vi "Labview_USB_I2C_AT24C02.vi"() -> ()   [LabVIEW 2010]
uses:
  Labview_USB_I2C_AM2321B/lib/labview_32bit/ControlI2C/Ginkgo_Driver.dll
panel:
  out "Flag(T:read;F:write)":bool=TRUE
  in  "Constant":T1={"DevType"=1, "DevIndex"=0, "I2CIndex"=0, "Addr"=0, "SubAddr"=0}
  in  "pInitConfig":T2={"MasterMode"=1, "ControlMode"=1, "AddrType"=7, "SubAddrWidth"=0, "Addr"=0, "@dummy control@"=0, "@dummy control@"=0, "ClockSpeed"=0}
  out "error out":errorcluster
  in  "Read":bool
  in  "Write":bool
  in  "Sub Addr(Hex)":u8 format="%x"
  in  "Slave Addr(Hex)":u8 format="%x"
  out "Read Data(Hex)":string
  in  "Channel Index":u16(ring) items=["0", "1"]
  in  "Speed":u32(ring)=800000 items=["800Kbps"=800000, "400Kbps"=400000, "200Kbps"=200000, "100Kbps"=100000, "50Kbps"=50000]
  in  "Write Data(Hex)":string
  in  "Device Index":u16(ring) items=["0", "1", "2", "3", "4", "5", "6", "7", "8", "9"]
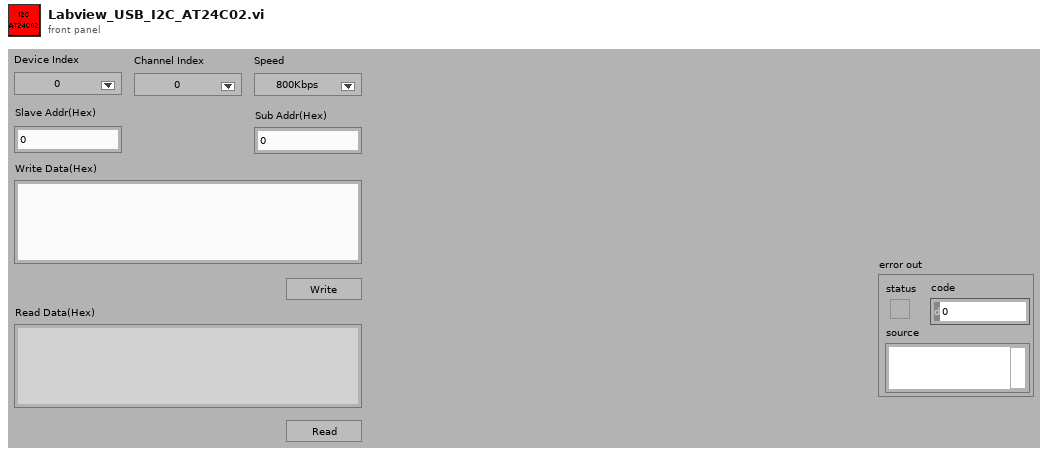
[diagram p1: front panel]
types:
  T1 = cluster{"DevType":i32, "DevIndex":i32, "I2CIndex":i32, "Addr":u16, "SubAddr":u32}
  T2 = cluster{"MasterMode":u8, "ControlMode":u8, "AddrType":u8, "SubAddrWidth":u8, "Addr":u16, "@dummy control@":i8, "@dummy control@":i8, "ClockSpeed":u32}
  T3 = enum16{"Init", "Write", "Read", "Idel", "Close", "Error"}
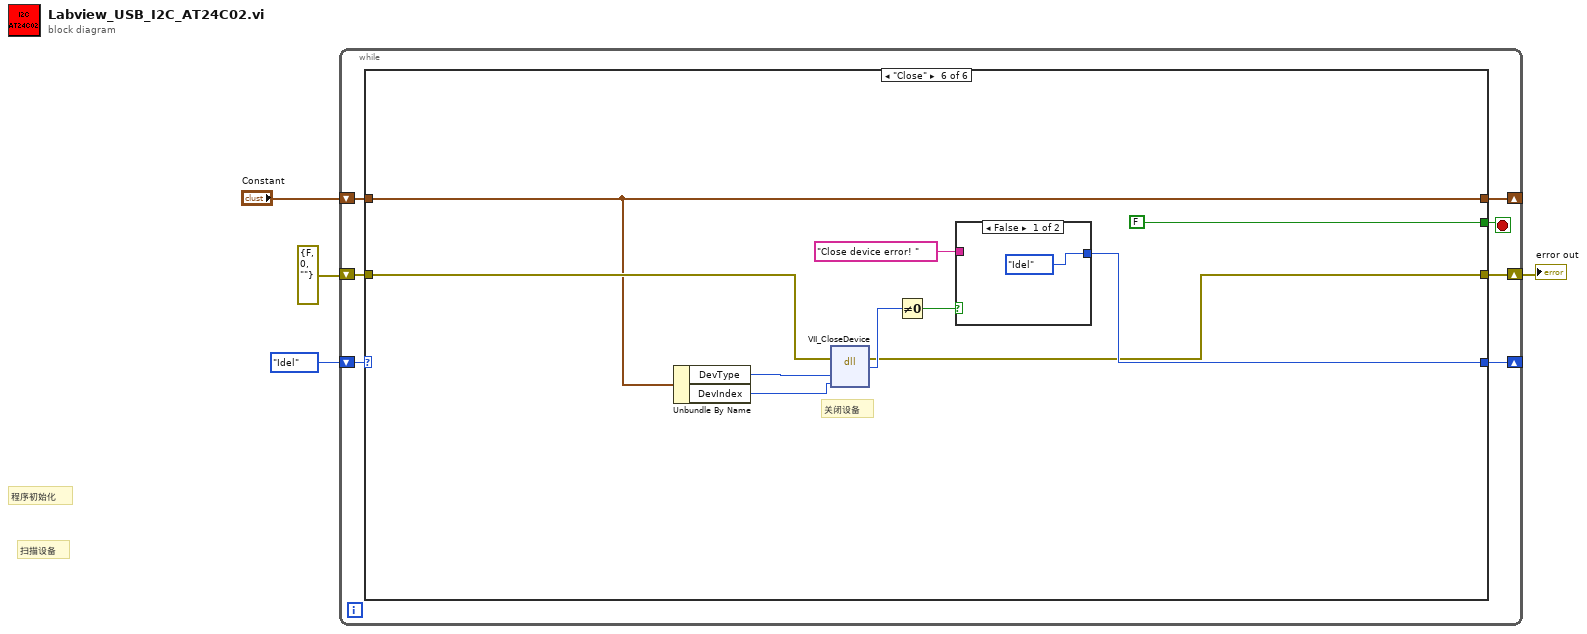
[diagram p0: block diagram]
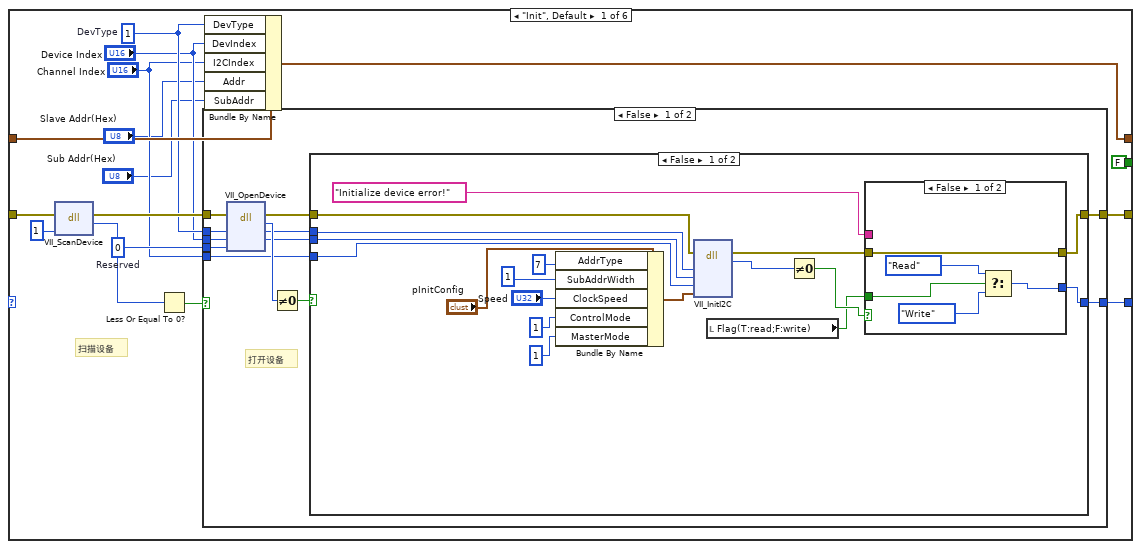
[diagram p2: hidden frame]
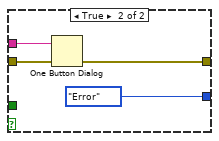
[diagram p3: hidden frame]
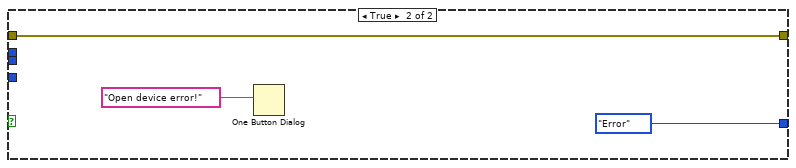
[diagram p4: hidden frame]
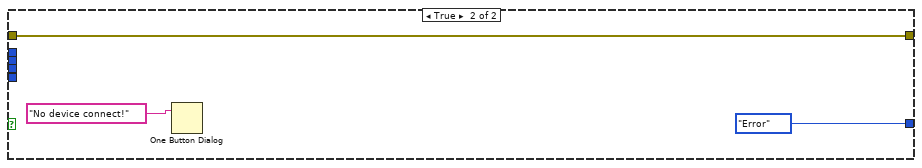
[diagram p5: hidden frame]
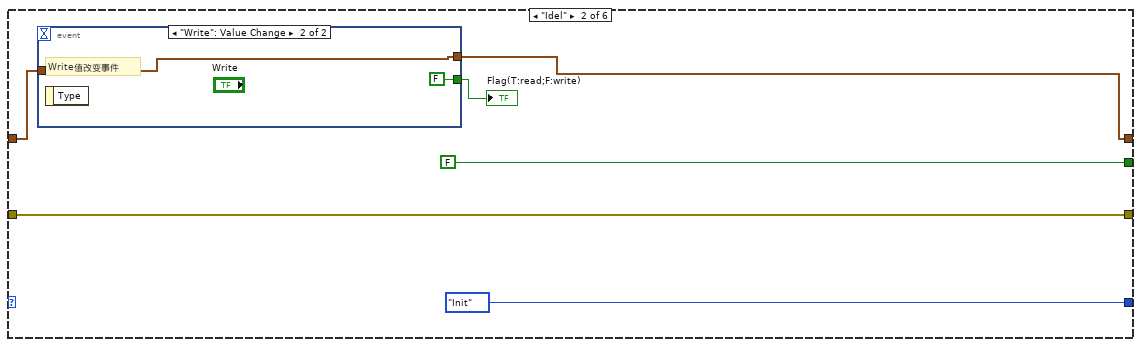
[diagram p6: hidden frame]
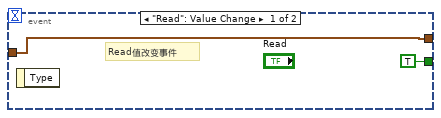
[diagram p7: hidden frame]
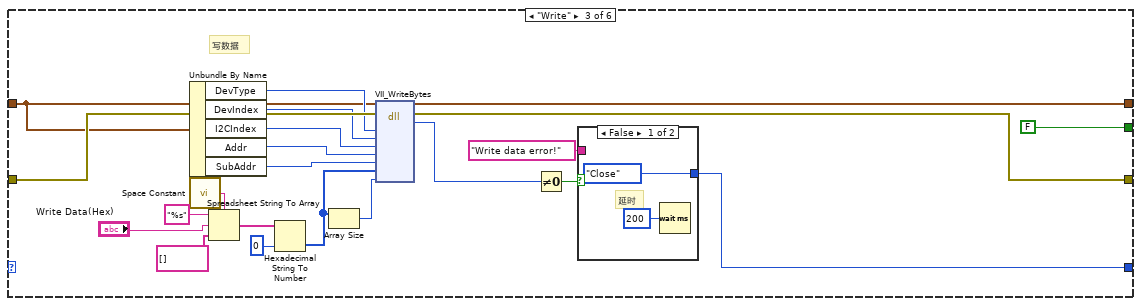
[diagram p8: hidden frame]
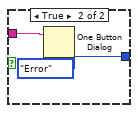
[diagram p9: hidden frame]
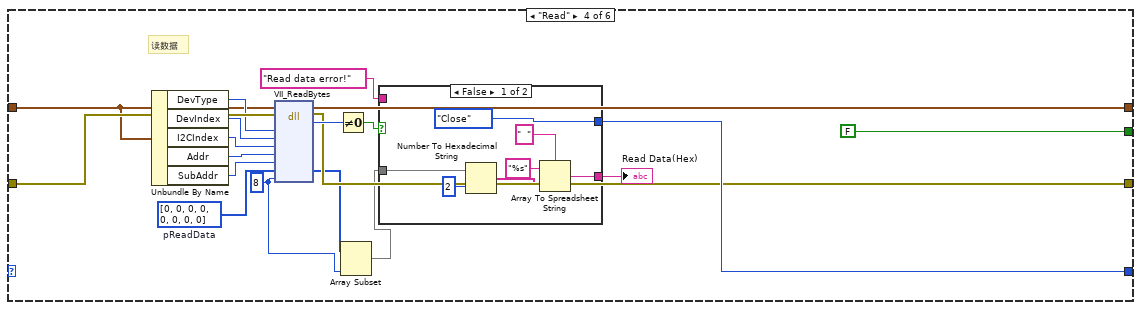
[diagram p10: hidden frame]
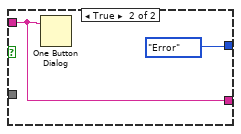
[diagram p11: hidden frame]
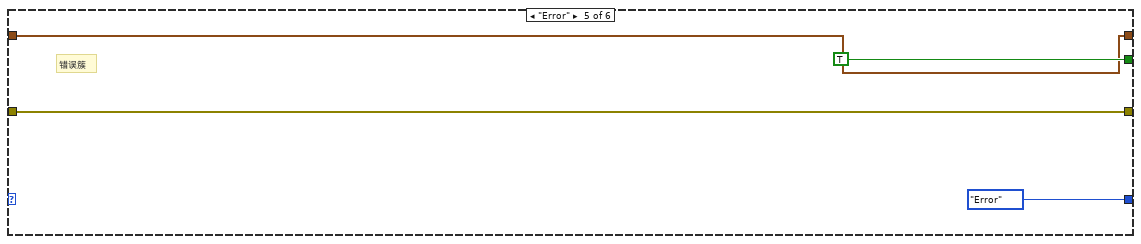
[diagram p12: hidden frame]
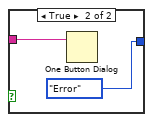
[diagram p13: hidden frame]
diagram:
  # "扫描设备"
  # "程序初始化"
  n1 = while {
    shift-right: [w11] -> _
    shift-left: T3."Idel" ("Enum") -> [w10]
    shift-right: [w8] -> w2
    shift-left: errorcluster {"status"=FALSE, "code"=0, "source"=""} ("error out") -> [w7]
    shift-right: [w5] -> _
    shift-left: "Constant" -> [w6]
    stop <- w9 stop-if-true
    n2 = case shown="\"Close\"" w10 {
      tunnel: [w19 T3."Init" ("Enum") w92 w115 T3."Error" ("Enum") w143] -> w11
      tunnel: [FALSE ("stop") FALSE ("stop") FALSE ("stop") FALSE ("stop") TRUE ("stop") FALSE ("stop")] -> w9
      tunnel: [w20 w76 w91 w114 w136 w142] -> w8
      tunnel: w7 -> [w21 w76 w101 w123 w136 w141]
      tunnel: w6 -> [w18 w75 w95 w113 w134 w140]
      tunnel: [w12 w74 w95 w113 w134 w140] -> w5
      frame "Init", Default {
        w22 = 0  # Reserved
        w17 = 1  # DevType
        # "扫描设备"
        n3 = dll-call lib="E:/Project/vt_ginkgo_examples/trunk/Labview/Ginkgo I2C/Labview_USB_I2C_AM2321B/lib/labview_32bit/ControlI2C/Ginkgo_Driver.dll" fn="VII_ScanDevice"(error in=w21, "NeedInit"=u8 1) -> (error out=w23:errorcluster, "return type"=w25:i32)  [unwired: 3 in, 1 out]
        n4 = Less Or Equal To 0?(x=w25) -> (x <= 0?=w24:bool)
        n5 = case shown="False" w24 {
          tunnel: [w33 T3."Error" ("Enum")] -> w19
          tunnel: w23 -> [w37 w70]
          tunnel: w22 -> [w36 _]
          tunnel: "Device Index" -> [w35 _]
          tunnel: w17 -> [w34 _]
          tunnel: [w29 w70] -> w20
          tunnel: "Channel Index" -> [w28 _]
          frame False {
            # "打开设备"
            n6 = dll-call lib="E:/Project/vt_ginkgo_examples/trunk/Labview/Ginkgo I2C/Labview_USB_I2C_AM2321B/lib/labview_32bit/ControlI2C/Ginkgo_Driver.dll" fn="VII_OpenDevice"(error in=w37, "DevType"=w34, "DevIndex"=w35, "Reserved"=w36) -> (error out=w32:errorcluster, "return type"=w38:i32, "DevType"=w31:i32, "DevIndex"=w30:i32)  [unwired: 3 in, 1 out]
            n7 = Not Equal To 0?(x=w38) -> (x != 0?=w39:bool)
            n8 = case shown="False" w39 {
              tunnel: [w46 T3."Error" ("Enum")] -> w33
              tunnel: w32 -> [w49 w67]
              tunnel: w31 -> [w48 _]
              tunnel: w30 -> [w47 _]
              tunnel: [w45 w67] -> w29
              tunnel: w28 -> [w44 _]
              frame False {
                n9 = Bundle By Name(cluster="pInitConfig", "AddrType"=u8 7, "SubAddrWidth"=u8 1, "ClockSpeed"="Speed", "ControlMode"=u8 1, "MasterMode"=u8 1) -> (w55:T2)
                n10 = dll-call lib="E:/Project/vt_ginkgo_examples/trunk/Labview/Ginkgo I2C/Labview_USB_I2C_AM2321B/lib/labview_32bit/ControlI2C/Ginkgo_Driver.dll" fn="VII_InitI2C"(error in=w49, "DevType"=w48, "DevIndex"=w47, "I2CIndex"=w44, "pInitConfig"=w55) -> (error out=w52:errorcluster, "return type"=w57:i32)  [unwired: 6 in, 1 out]
                n11 = local read "Flag(T:read;F:write)"() -> (w40:bool)
                n12 = Not Equal To 0?(x=w57) -> (x != 0?=w56:bool)
                n13 = case shown="False" w56 {
                  tunnel: "Initialize device error!" ("message") -> [_ w65]
                  tunnel: [w58 T3."Error" ("Enum")] -> w46
                  tunnel: w52 -> [w62 w63]
                  tunnel: [w62 w63] -> w45
                  tunnel: w40 -> [w61 _]
                  frame False {
                    n14 = Select(t=T3."Read" ("Enum"), s=w61, f=T3."Write" ("Enum")) -> (s? t:f=w58:T3)
                  }
                  frame True {
                    n15 = One Button Dialog(message=w65) -> ()  [unwired: 1 in, 1 out]
                  }
                }
              }
              frame True {
                n16 = One Button Dialog(message="Open device error!") -> ()  [unwired: 1 in, 1 out]
              }
            }
          }
          frame True {
            n17 = One Button Dialog(message="No device connect!") -> ()  [unwired: 1 in, 1 out]
          }
        }
        n18 = Bundle By Name(cluster=w18, "DevType"=w17, "DevIndex"="Device Index", "I2CIndex"="Channel Index", "Addr"="Slave Addr(Hex)", "SubAddr"="Sub Addr(Hex)") -> (w12:T1)
      }
      frame "Idel" {
        n19 = event shown="[1] \"Write\": Value Change" {
          selector: _ -> [_ _]
          dyn-events: _ -> [_ _]
          timeout: _ -> [_ _]
          tunnel: w75 -> [w79 w81]
          tunnel: [w79 w81] -> w74
          tunnel: [TRUE ("Read") FALSE ("Read")] -> w72
          event "Read": Value Change {
            # "Read值改变事件"
            n20 = event-data() -> ()  [unwired: 1 in, 1 out]
          }
          event "Write": Value Change {
            # "Write值改变事件"
            n21 = event-data() -> ()  [unwired: 1 in, 1 out]
          }
        }
        "Flag(T:read;F:write)" <- w72
      }
      frame "Write" {
        # "写数据"
        n22 = Unbundle By Name(w95) -> ("DevType"=w100:i32, "DevIndex"=w99:i32, "I2CIndex"=w98:i32, "Addr"=w97:u16, "SubAddr"=w96:u32)
        n23 = call <vilib>:"Space Constant.vi"() -> ("String"=w84:string)
        n24 = Spreadsheet String To Array(delimiter (Tab)=w84, format string="%s", spreadsheet string="Write Data(Hex)", array type (2D Dbl)=string[] []) -> (array=w87:string[])
        n25 = Hexadecimal String To Number(string=w87, default (0uL)=u8 0 ("default (0 U32)")) -> (number=w82:u8[])  [unwired: 1 in, 1 out]
        n26 = Array Size(array=w82) -> (size(s)=w89:i32)
        n27 = dll-call lib="E:/Project/vt_ginkgo_examples/trunk/Labview/Ginkgo I2C/Labview_USB_I2C_AM2321B/lib/labview_32bit/ControlI2C/Ginkgo_Driver.dll" fn="VII_WriteBytes"(error in=w101, "DevType"=w100, "DevIndex"=w99, "I2CIndex"=w98, "Addr"=w97, "SubAddr"=w96, "pWriteData"=w82, "Len"=w89) -> (error out=w91:errorcluster, "return type"=w93:i32)  [unwired: 9 in, 1 out]
        n28 = Not Equal To 0?(x=w93) -> (x != 0?=w90:bool)
        n29 = case shown="False" w90 {
          tunnel: "Write data error!" ("message") -> [_ w106]
          tunnel: [T3."Close" ("Enum") T3."Error" ("Enum")] -> w92
          frame False {
            # "延时"
            n30 = Wait (ms)(milliseconds to wait=u32 200) -> ()  [unwired: 1 out]
          }
          frame True {
            n31 = One Button Dialog(message=w106) -> ()  [unwired: 1 in, 1 out]
          }
        }
      }
      frame "Read" {
        w110 = u8[] [0, 0, 0, 0, 0, 0, 0, 0]  # pReadData
        w108 = u16 8 ("Len")
        # "读数据"
        n32 = Unbundle By Name(w113) -> ("DevType"=w122:i32, "DevIndex"=w121:i32, "I2CIndex"=w120:i32, "Addr"=w119:u16, "SubAddr"=w118:u32)
        n33 = dll-call lib="E:/Project/vt_ginkgo_examples/trunk/Labview/Ginkgo I2C/Labview_USB_I2C_AM2321B/lib/labview_32bit/ControlI2C/Ginkgo_Driver.dll" fn="VII_ReadBytes"(error in=w123, "DevType"=w122, "DevIndex"=w121, "I2CIndex"=w120, "Addr"=w119, "SubAddr"=w118, "pReadData"=w110, "Len"=w108) -> (error out=w114:errorcluster, "return type"=w117:i32, "pReadData"=w109:u8[])  [unwired: 8 in, 1 out]
        n34 = Not Equal To 0?(x=w117) -> (x != 0?=w112:bool)
        n35 = Array Subset(array=w109, length=w108) -> (w107:u8[])  [unwired: 1 in]
        n36 = case shown="False" w112 {
          tunnel: "Read data error!" ("message") -> [_ w132]
          tunnel: [T3."Close" ("Enum") T3."Error" ("Enum")] -> w115
          tunnel: w107 -> [w126 _]
          tunnel: [w125 w132] -> w111
          frame False {
            n37 = Number To Hexadecimal String(1:i16 2 ("width (-)"), 2:w126) -> (0:w128:string[])
            n38 = Array To Spreadsheet String(delimiter (Tab)="  ", array=w128, 3:"%s" ("format string")) -> (spreadsheet string=w125:string)
          }
          frame True {
            n39 = One Button Dialog(message=w132) -> ()  [unwired: 1 in, 1 out]
          }
        }
        "Read Data(Hex)" <- w111
      }
      frame "Error" {
        # "错误簇"
      }
      frame "Close" {
        # "关闭设备"
        n40 = Unbundle By Name(w140) -> ("DevType"=w139:i32, "DevIndex"=w138:i32)
        n41 = dll-call lib="E:/Project/vt_ginkgo_examples/trunk/Labview/Ginkgo I2C/Labview_USB_I2C_AM2321B/lib/labview_32bit/ControlI2C/Ginkgo_Driver.dll" fn="VII_CloseDevice"(error in=w141, "DevType"=w139, "DevIndex"=w138) -> (error out=w142:errorcluster, "return type"=w145:i32)  [unwired: 4 in, 1 out]
        n42 = Not Equal To 0?(x=w145) -> (x != 0?=w144:bool)
        n43 = case shown="False" w144 {
          tunnel: "Close device error! " ("message") -> [_ w150]
          tunnel: [T3."Idel" ("Enum") T3."Error" ("Enum")] -> w143
          frame False {
          }
          frame True {
            n44 = One Button Dialog(message=w150) -> ()  [unwired: 1 in, 1 out]
          }
        }
      }
    }
  }
  "error out" <- w2
